vi "Tracking Phaco.vi"(5 "Trajectory Cluster":T3, 6 "OCT Z PID Gains":cluster{"Kp":dbl, "Kd":dbl, "Ki":dbl}={"Kp"=0.0003, "Kd"=0.0001, "Ki"=0.01}, 7 "Eye Model Cluster":T2={"X Grid"=[], "Y Grid"=[], "Za_true Surf"=[], "Iris Center"=[], "Zp_true Surf"=[], "Pinv"=[[1.0, 0.0], [0.0, 1.0]], "za_true"=5.0, "za_work"=1.0, "zp_work"=-1.0, "zp_true"=-5.0}, 8 "error in":errorcluster, 9 "OCT Prev Posit":dbl, 10 "Resume Index":i32, 11 "FPGA VI Reference In":refnum<k20>) -> (0 "error out":errorcluster, 1 "OCT Last Posit":dbl, 2 "Leave Index":i32, 3 "FPGA VI Reference Out":refnum<k20>)   [LabVIEW 2016]
uses:
  <vilib>/Analysis/Matrix/Datatypes/RealMatrix.ctl
  <vilib>/Platform/TimedLoop/XDataNode/timing_clust.ctl
  <vilib>/Platform/TimedLoop/XDataNode/nitl_modes.ctl
  <vilib>/Platform/TimedLoop/XDataNode/wakeup.ctl
  Subsystems/Global Variables.vi
  <vilib>/platform/TimedLoop/XDataNode/XDataNode.xnode
  <vilib>/Platform/TimedLoop/XDataNode/XDNodeRunTimeDep.lvlib
  Library/KevinLibraryAll/labview/KevLib01.lvlib
  <vilib>/Analysis/Matrix/NI_Matrix.lvlib
panel:
  out "In Servo Loop":bool
  out "PC z Displacement":dbl
  out "Speed Schedule":dbl
  out "joint limits":dbl[][](array[numeric])=[[-10.0, 35.0], [-35.0, 35.0], [0.1, 10.0], [-40.0, 40.0]]
  out "Vac Extremum":dbl[](array[numeric])
  out "z Dist Thld":dbl[](array[numeric])
  out "z Rot Axis":dbl
  out "Deform Array":dbl[](array[numeric])=[1.0, 1.0, 1.0, 0.0, 0.0, 0.0, 0.0, 0.0, 0.0]
  out "Speed Override":u16(ring)=3 items=["4x", "3x", "2x", "1x", "0.5x", "0.2x", "0.1x", "PAUSE"]
  out "Loading Finished":bool
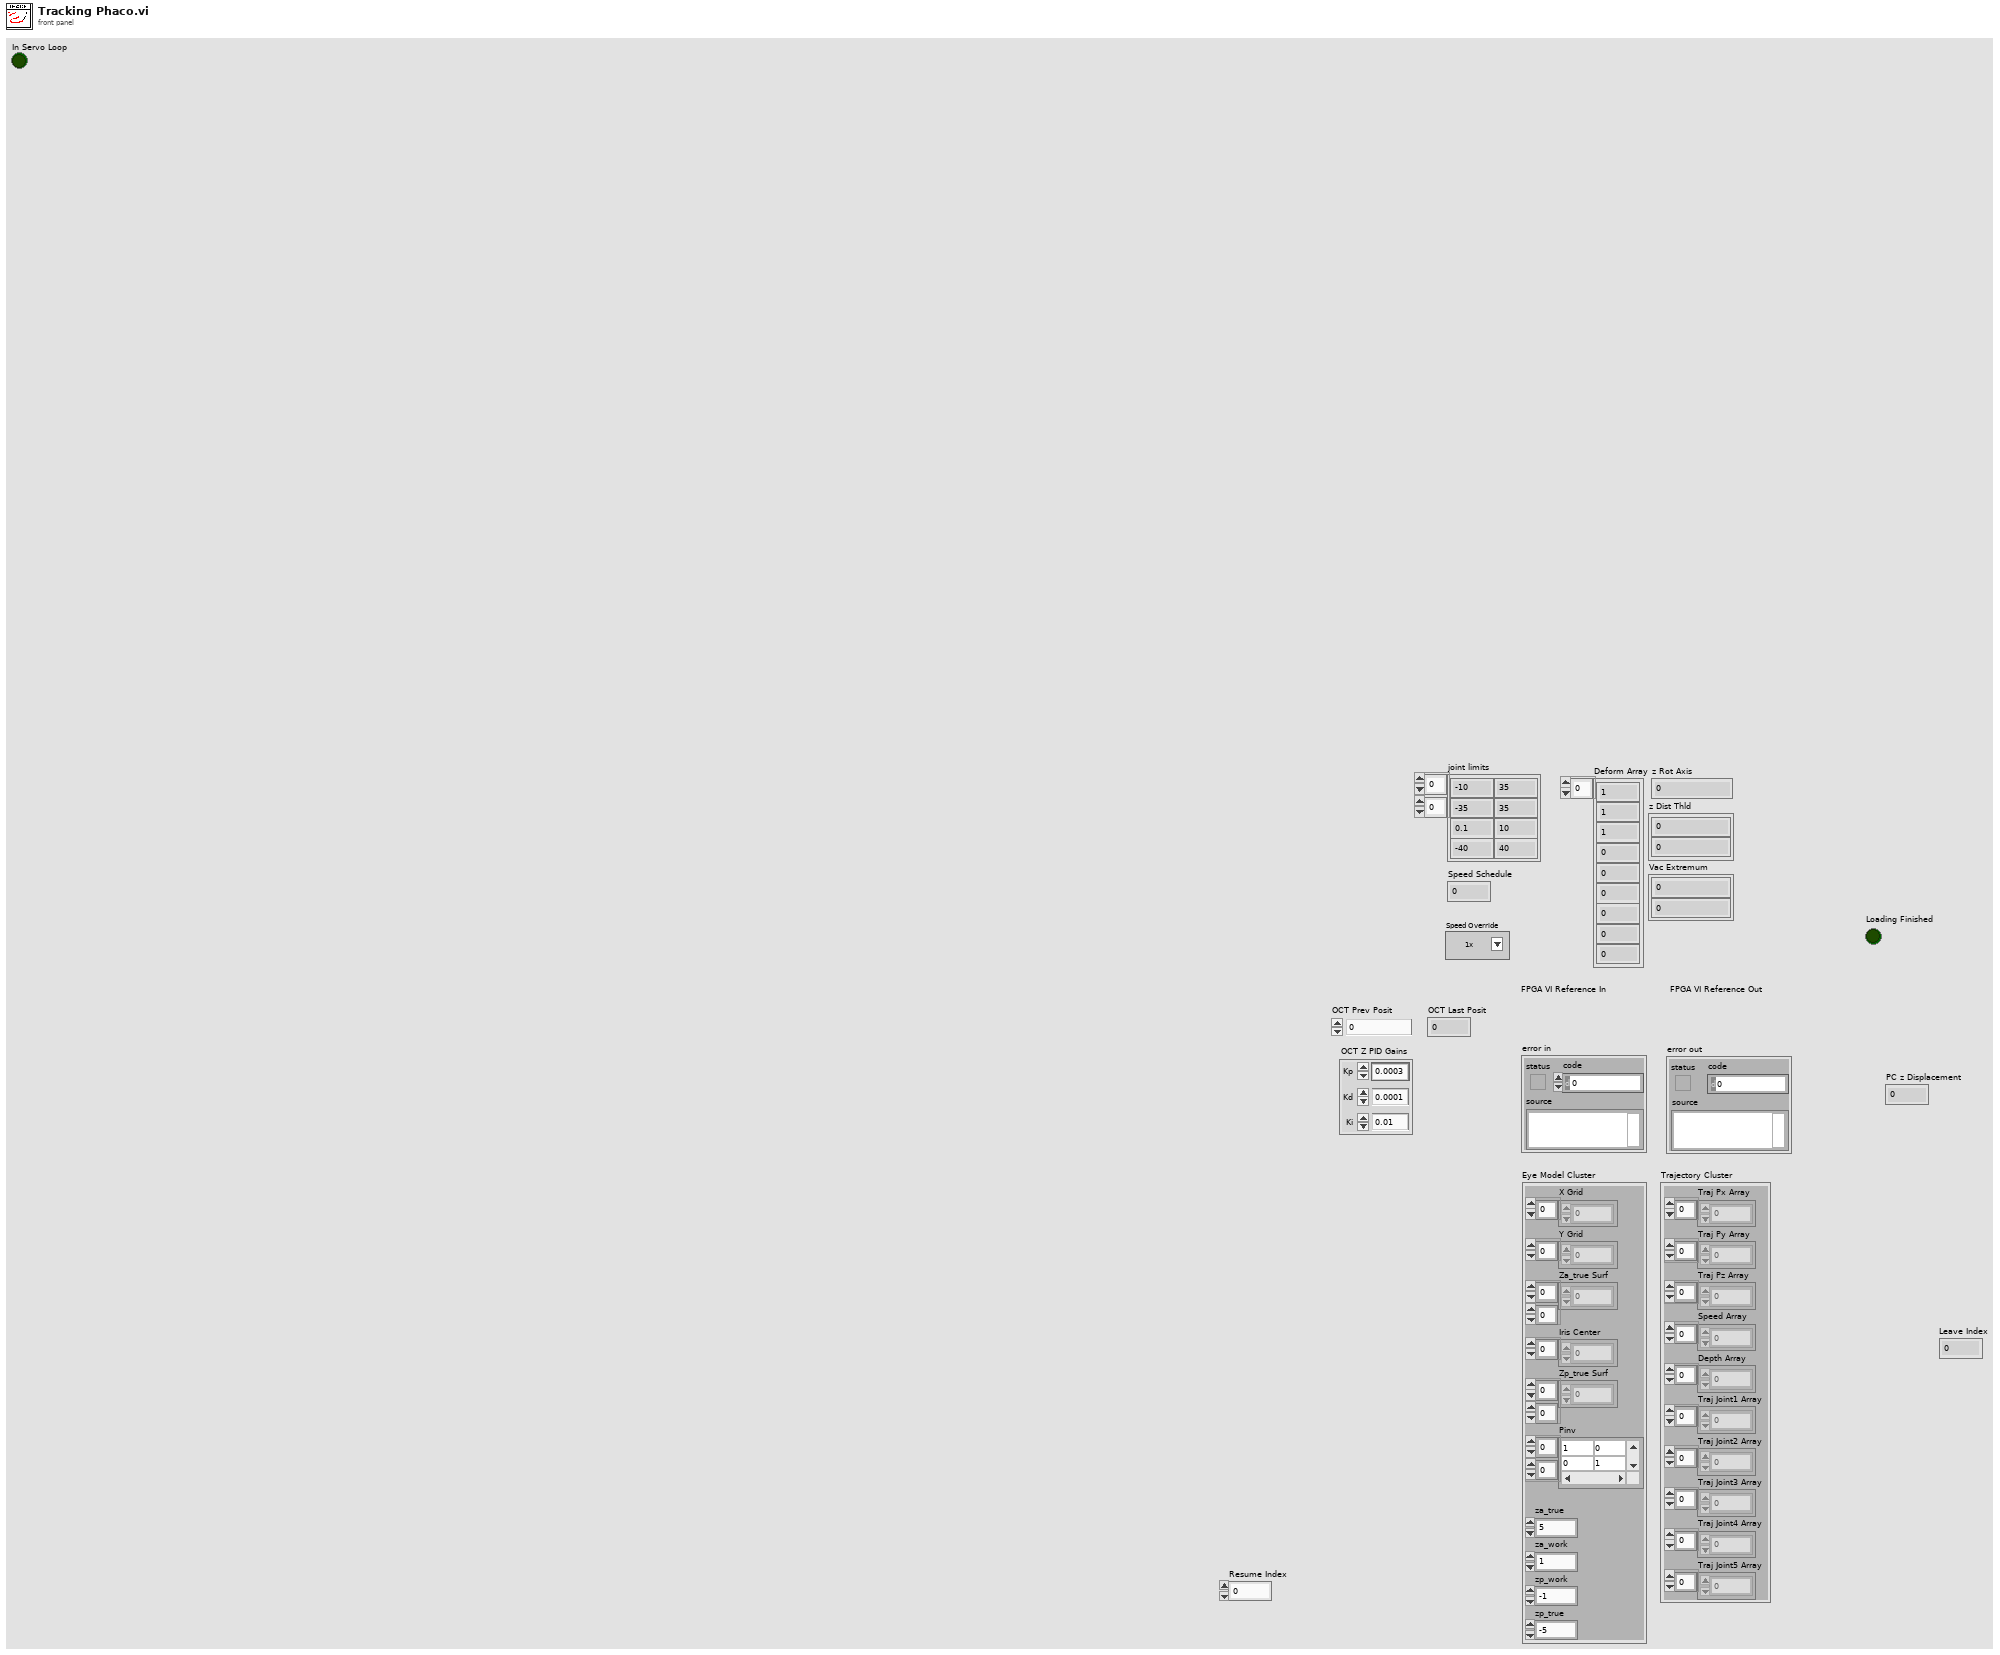
[diagram p1: front panel]
types:
  T1 = typedef "NI_Matrix.lvlib/RealMatrix.ctl" = dbl[][]
  T2 = cluster{"X Grid":dbl[], "Y Grid":dbl[], "Za_true Surf":dbl[][], "Iris Center":dbl[], "Zp_true Surf":dbl[][], "Pinv":T1, "za_true":dbl, "za_work":dbl, "zp_work":dbl, "zp_true":dbl}
  T3 = cluster{"Traj Px Array":dbl[], "Traj Py Array":dbl[], "Traj Pz Array":dbl[], "Speed Array":dbl[], "Depth Array":dbl[], "Traj Joint1 Array":dbl[], "Traj Joint2 Array":dbl[], "Traj Joint3 Array":dbl[], "Traj Joint4 Array":dbl[], "Traj Joint5 Array":dbl[]}
  T4 = typedef "XDNodeRunTimeDep.lvlib/timing_clust.ctl" = cluster{"Expected End [f-1]":u64, "Actual End [f-1]":u64, "Finished Late? [f-1]":bool, "Expected End [i-1]":u64, "Actual End [i-1]":u64, "Finished Late? [i-1]":bool, "Expected Start [i]":u64, "Actual Start [i]":u64, "Expected Start [f]":u64, "Actual Start [f]":u64, "Source Name":string, "Structure Name":string, "Period":i64, "Deadline":i64, "Offset":i64, "Start":i64, "Priority":i32, "Timeout":i32, "Mode":T5, "Wakeup Reason":T6, "Error":errorcluster, "Source Type":string, "Secondary Source Type":string, "Global End Time":u64, "Global Start Time":u64, "Frame Duration":u64, "Iteration Duration":u64, "Assigned CPU":i32, "I/O Scan Engine Mode":u32}
  T5 = typedef "XDNodeRunTimeDep.lvlib/nitl_modes.ctl" = enum32{"No Change", "Process missed periods, maintain original phase", "Discard missed periods, maintain original phase", "Process missed periods, ignore original phase", "Discard missed periods, ignore original phase"}
  T6 = typedef "XDNodeRunTimeDep.lvlib/wakeup.ctl" = enum32{"Normal", "Aborted", "Asynchronous wakeup", "Timing source error", "Timed loop error", "Timeout"}
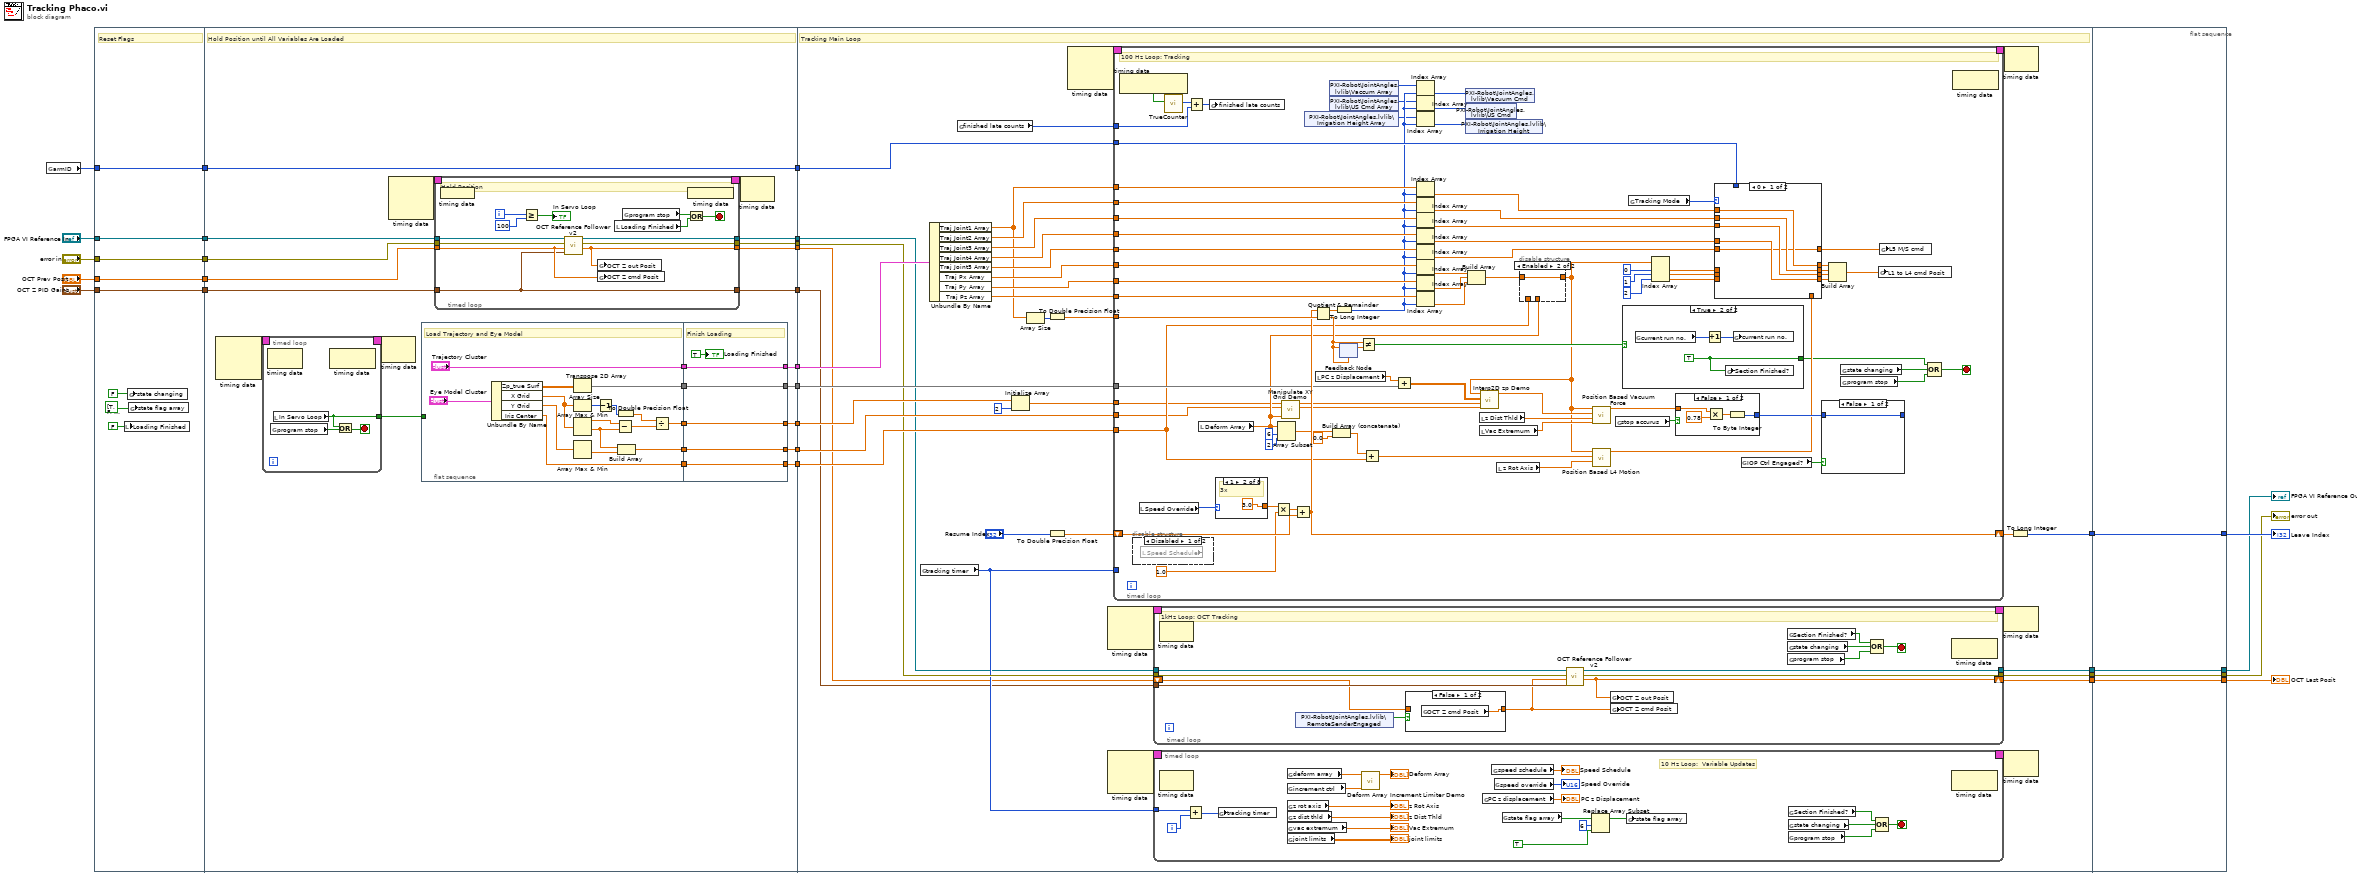
[diagram p0: block diagram]
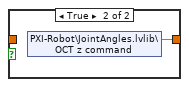
[diagram p2: hidden frame]
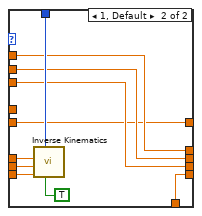
[diagram p3: hidden frame]
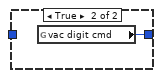
[diagram p5: hidden frame]
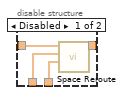
[diagram p6: hidden frame]
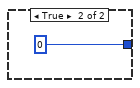
[diagram p7: hidden frame]
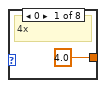
[diagram p8: hidden frame]
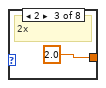
[diagram p9: hidden frame]
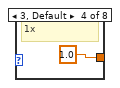
[diagram p10: hidden frame]
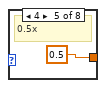
[diagram p11: hidden frame]
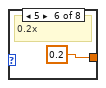
[diagram p12: hidden frame]
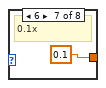
[diagram p13: hidden frame]
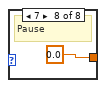
[diagram p14: hidden frame]
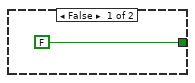
[diagram p15: hidden frame]
diagram:
  n1 = global read "Global Variables.vi" "armID"() -> (w14:i32)
  n2 = flat-sequence {
    tunnel: [w34] -> w28
    tunnel: "FPGA VI Reference In" -> [w34]
    tunnel: "error in" -> [w33]
    tunnel: [w33] -> w25
    tunnel: w14 -> [w32]
    tunnel: [w32] -> w16
    tunnel: [w30] -> w13
    tunnel: "OCT Prev Posit" -> [w30]
    tunnel: [w29] -> w11
    tunnel: "OCT Z PID Gains" -> [w29]
    tunnel: w28 -> [w47]
    tunnel: w25 -> [w46]
    tunnel: [w42] -> w24
    tunnel: [w60] -> w23
    tunnel: [w59] -> w22
    tunnel: [w58] -> w21
    tunnel: [w57] -> w19
    tunnel: [w56] -> w18
    tunnel: [w50] -> w17
    tunnel: w16 -> [w50]
    tunnel: [w43] -> w15
    tunnel: w13 -> [w45]
    tunnel: w11 -> [w44]
    tunnel: [w38] -> w9
    tunnel: [w37] -> w8
    tunnel: w24 -> [w123]
    tunnel: w23 -> [w137]
    tunnel: w22 -> [w129]
    tunnel: w21 -> [w138]
    tunnel: w19 -> [w130]
    tunnel: w18 -> [w131]
    tunnel: w17 -> [w126]
    tunnel: w15 -> [w120]
    tunnel: w9 -> [w119]
    tunnel: w8 -> [w118]
    tunnel: [w134] -> w6
    tunnel: [w122] -> w5
    tunnel: [w117] -> w4
    tunnel: [w107] -> w3
    tunnel: [w315] -> w7
    tunnel: [w316] -> w1
    tunnel: [w317] -> w20
    tunnel: w6 -> [w317]
    tunnel: w5 -> [w316]
    tunnel: w4 -> [w315]
    tunnel: w3 -> [w314]
    tunnel: [w314] -> w2
    frame #0 {
      # "Reset Flags"
      n3 = local write "Loading Finished"(FALSE ("Loading Finished")) -> ()
      n4 = global write "Global Variables.vi" "state changing"(FALSE ("state changing")) -> ()
      n5 = global write "Global Variables.vi" "state flag array"(bool[] [TRUE, FALSE, FALSE, FALSE, FALSE, FALSE, FALSE, FALSE, FALSE] ("state flag array")) -> ()
    }
    frame #1 {
      # "Hold Position until All Variables Are Loaded"
      n6 = node-c288() -> (w41:T4)  [unwired: 3 in]
      n7 = timed-loop {
        timing: w41 -> [_]
        timing-out: [_] -> w40
        tunnel: [w61] -> w39
        stop <- w63 stop-if-true
        n8 = node-c288() -> ()  [unwired: 1 in, 1 out]
        n9 = global read "Global Variables.vi" "program stop"() -> (w62:bool)
        n10 = local read "In Servo Loop"() -> (w61:bool)
        n11 = node-c288() -> ()  [unwired: 1 in, 1 out]
        n12 = Or(x=w61, y=w62) -> (x .or. y?=w63:bool)
      }
      n13 = node-c288(w40) -> ()  [unwired: 1 out]
      n14 = node-c288() -> (w49:T4)  [unwired: 3 in]
      n15 = flat-sequence {
        tunnel: [w87] -> w55
        tunnel: [w100] -> w54
        tunnel: [w99] -> w53
        tunnel: [w86] -> w52
        tunnel: ["Trajectory Cluster"] -> w51
        tunnel: w39 -> [_]
        tunnel: [w104] -> w58
        tunnel: [w105] -> w59
        tunnel: [w106] -> w60
        tunnel: w55 -> [w106]
        tunnel: w54 -> [w105]
        tunnel: w53 -> [w104]
        tunnel: w52 -> [w102]
        tunnel: [w102] -> w57
        tunnel: [w101] -> w56
        tunnel: w51 -> [w101]
        frame #0 {
          # "Load Trajectory and Eye Model"
          n16 = Unbundle By Name("Eye Model Cluster") -> ("Zp_true Surf"=w88:dbl[][], "X Grid"=w89:dbl[], "Y Grid"=w98:dbl[], "Iris Center"=w86:dbl[])
          n17 = Transpose 2D Array(2D array=w88) -> (transposed array=w87:dbl[][])
          n18 = Array Size(array=w89) -> (size(s)=w97:i32)
          n19 = Array Max & Min(array=w89) -> (max value=w95:dbl, min value=w96:dbl)  [unwired: 2 out]
          n20 = Array Max & Min(array=w98) -> (min value=w94:dbl)  [unwired: 3 out]
          n21 = Decrement(x=w97) -> (x-1=w92:i32)
          n22 = Subtract(x=w95, y=w96) -> (x-y=w91:dbl)
          n23 = To Double Precision Float(number=w92) -> (double precision float=w93:dbl)
          n24 = Build Array(w96, w94) -> (w99:dbl[])
          n25 = Divide(x=w93, y=w91) -> (x/y=w100:dbl)
        }
        frame #1 {
          # "Finish Loading"
          "Loading Finished" <- TRUE ("Loading Finished")
        }
      }
      n26 = timed-loop {
        timing: w49 -> [_]
        timing-out: [_] -> w48
        tunnel: [w71] -> w37
        tunnel: [w68] -> w43
        tunnel: [w72] -> w42
        tunnel: w47 -> [w74]
        tunnel: w46 -> [w73]
        tunnel: w44 -> [w69]
        tunnel: w45 -> [w70]
        tunnel: [w69] -> w38
        i -> [w77]
        stop <- w80 stop-if-true
        # "Hold Position"
        n27 = node-c288 ("Output Node")() -> ()  [unwired: 1 in]
        n28 = Greater Or Equal?(x=w77, y=100) -> (x >= y?=→"In Servo Loop":bool)
        n29 = call "OCT Reference Follower v2.vi"("OCT Z PID Gains"=w69, "OCT  Z cmd Posit [mm]"=w70, "error in"=w73, "FPGA VI Reference In"=w74) -> ("OCT  Z out Posit [mm]"=w71:dbl, "error out"=w72:errorcluster, "FPGA VI Reference Out"=w68:refnum<k20>)  [unwired: 5 in]
        n30 = global write "Global Variables.vi" "OCT Z out Posit"(w71) -> ()
        n31 = global write "Global Variables.vi" "OCT Z cmd Posit"(w70) -> ()
        n32 = local read "Loading Finished"() -> (w79:bool)
        n33 = global read "Global Variables.vi" "program stop"() -> (w78:bool)
        n34 = Or(x=w78, y=w79) -> (x .or. y?=w80:bool)
        n35 = node-c288() -> ()  [unwired: 1 out]
      }
      n36 = node-c288(w48) -> ()  [unwired: 1 out]
    }
    frame #2 {
      # "Tracking Main Loop"
      n37 = global read "Global Variables.vi" "tracking timer"() -> (w121:i32)
      n38 = Unbundle By Name(w131) -> ("Traj Joint1 Array"=w110:dbl[], "Traj Joint2 Array"=w116:dbl[], "Traj Joint3 Array"=w115:dbl[], "Traj Joint4 Array"=w114:dbl[], "Traj Joint5 Array"=w111:dbl[], "Traj Px Array"=w113:dbl[], "Traj Py Array"=w136:dbl[], "Traj Pz Array"=w132:dbl[])
      n39 = global read "Global Variables.vi" "finished late counts"() -> (w141:u16)
      n40 = Initialize Array(w129, 2 ("dimension size")) -> (w127:dbl[])
      n41 = Array Size(array=w110) -> (size(s)=w109:i32)
      n42 = To Double Precision Float(number=w109) -> (double precision float=w112:dbl)
      n43 = To Double Precision Float(number="Resume Index") -> (double precision float=w133:dbl)
      n44 = node-c288() -> (w143:T4)  [unwired: 3 in]
      n45 = node-c288() -> (w125:T4)  [unwired: 3 in]
      n46 = node-c288() -> (w140:T4)  [unwired: 3 in]
      n47 = timed-loop {
        timing: w143 -> [_]
        timing-out: [_] -> w142
        tunnel: w113 -> [w269]
        tunnel: w136 -> [w268]
        tunnel: w132 -> [w263]
        tunnel: w141 -> [w264]
        shift-right: [w250] -> w135
        shift-left: w133 -> [w253]
        tunnel: w137 -> [w246]
        tunnel: w127 -> [w243]
        tunnel: w138 -> [w242]
        tunnel: w112 -> [w252]
        tunnel: w130 -> [w245]
        tunnel: w121 -> [_]
        tunnel: w126 -> [w213]
        tunnel: w110 -> [w210]
        tunnel: w116 -> [w211]
        tunnel: w115 -> [w212]
        tunnel: w114 -> [w203]
        tunnel: w111 -> [w202]
        stop <- w196 stop-if-true
        # "100 Hz Loop: Tracking"
        n48 = node-c288() -> (w267:bool)  [unwired: 1 in]
        n49 = disable-structure shown="Disabled" {
          frame Disabled {
            n50 = local read "Speed Schedule"() -> ()  [unwired: 1 out]
          }
          frame Enabled {
          }
        }
        n51 = local read "Speed Override"() -> (w255:u16)
        n52 = call "TrueCounter.vi"("True?"=w267) -> ("True Count"=w265:u16)  [unwired: 10 in]
        n53 = Add(x=w265, y=w264) -> (x+y=w266:u16)
        n54 = local read "Deform Array"() -> (w244:dbl[])
        n55 = global write "Global Variables.vi" "finished late counts"(w266) -> ()
        n56 = case shown="1" w255 {
          tunnel: [4.0 ("y") 3.0 ("y") 2.0 ("y") 1.0 ("y") 0.5 ("y") 0.2 ("y") 0.1 ("y") 0.0 ("y")] -> w254
          frame 0 {
            # "4x"
          }
          frame 1 {
            # "3x"
          }
          frame 2 {
            # "2x"
          }
          frame 3, Default {
            # "1x"
          }
          frame 4 {
            # "0.5x"
          }
          frame 5 {
            # "0.2x"
          }
          frame 6 {
            # "0.1x"
          }
          frame 7 {
            # "Pause"
          }
        }
        n57 = Multiply(x=w254, y=1.0) -> (x*y=w256:dbl)
        n58 = Array Subset(array=w244, index=6, length=2) -> (w229:dbl[])
        n59 = call "Manipulate XY Grid Demo.vi"("Deform Array"=w244, "XY Grid min In"=w242, "XY Quant. Fact. In"=w243) -> ("XY Grid min Out"=w224:dbl[], "XY Quant. Fact. Out"=w225:dbl[])  [unwired: 7 in]
        n60 = Add(x=w256, y=w253) -> (x+y=w250:dbl)
        n61 = shared-variable "PXI-Robot\\JointAngles.lvlib\\Irrigation Height Array"() -> (w194:i32[])  [unwired: 1 in, 1 out]
        n62 = Quotient & Remainder(x=w250, y=w252) -> (x-y*floor(x/y)=w251:dbl, floor(x/y)=w247:dbl)
        n63 = local read "PC z Displacement"() -> (w232:dbl)
        n64 = shared-variable "PXI-Robot\\JointAngles.lvlib\\Vaccum Array"() -> (w193:i32[])  [unwired: 1 in, 1 out]
        n65 = shared-variable "PXI-Robot\\JointAngles.lvlib\\US Cmd Array"() -> (w192:i32[])  [unwired: 1 in, 1 out]
        n66 = Build Array (concatenate)(w229, 0.0) -> (w228:dbl[])
        n67 = To Long Integer(number=w251) -> (32bit integer=w195:i32)
        n68 = feedback-in #1(w247) -> ()
        n69 = feedback #1(w247) -> (w249:dbl)
        n70 = Not Equal?(x=w247, y=w249) -> (x != y?=w248:bool)
        n71 = Add(x=w228, y=w245) -> (x+y=w219:dbl[])
        n72 = Add(x=w232, y=w246) -> (x+y=w226:dbl[][])
        n73 = Index Array(array=w193, index=w195) -> (element=w189:i32)
        n74 = Index Array(array=w192, index=w195) -> (element=w191:i32)
        n75 = Index Array(array=w194, index=w195) -> (element=w190:i32)
        n76 = Index Array(array=w210, index=w195) -> (element=w208:dbl)
        n77 = Index Array(array=w211, index=w195) -> (element=w207:dbl)
        n78 = Index Array(array=w212, index=w195) -> (element=w206:dbl)
        n79 = Index Array(array=w203, index=w195) -> (element=w201:dbl)
        n80 = Index Array(array=w202, index=w195) -> (element=w200:dbl)
        n81 = Index Array(array=w269, index=w195) -> (element=w259:dbl)
        n82 = Index Array(array=w268, index=w195) -> (element=w258:dbl)
        n83 = Index Array(array=w263, index=w195) -> (element=w257:dbl)
        n84 = shared-variable "PXI-Robot\\JointAngles.lvlib\\Vacuum Cmd"(w189) -> ()  [unwired: 1 in, 1 out]
        n85 = shared-variable "PXI-Robot\\JointAngles.lvlib\\US Cmd"(w191) -> ()  [unwired: 1 in, 1 out]
        n86 = shared-variable "PXI-Robot\\JointAngles.lvlib\\Irrigation Height"(w190) -> ()  [unwired: 1 in, 1 out]
        n87 = Build Array(w259, w258, w257) -> (w241:dbl[])
        n88 = local read "z Dist Thld"() -> (w222:dbl[])
        n89 = local read "Vac Extremum"() -> (w221:dbl[])
        n90 = local read "z Rot Axis"() -> (w218:dbl)
        n91 = disable-structure shown="Enabled" {
          disable-tunnel: w245 -> [w290 _]
          disable-tunnel: w244 -> [w289 _]
          disable-tunnel: w241 -> [w288 w291]
          disable-tunnel: [w287 w291] -> w217
          frame Disabled {
            n92 = call "Space Reroute.vi"("Deform Array"=w289, "Pivot Pt"=w290, "Nominal Traj Pt"=w288) -> ("Reroute Traj Pt"=w287:dbl[])  [unwired: 8 in]
          }
          frame Enabled {
          }
        }
        n93 = call "Interp2D zp Demo.vi"("XY Grid min"=w224, "XY Quantization Factor"=w225, "Zp array"=w226, "Tip Position"=w217) -> ("zp"=w223:dbl)  [unwired: 7 in]
        n94 = call "Position Based Vacuum Force.vi"("vac_bnd"=w221, "z_thld"=w222, "current zp"=w223, "tip position"=w217) -> ("vacf (%)"=w220:dbl)  [unwired: 7 in]
        n95 = call "Position Based L4 Motion.vi"("Assign z"=w218, "Iris Center"=w219, "Tip Position"=w217) -> ("L4 Motion [deg]"=w205:dbl)  [unwired: 8 in]
        n96 = global read "Global Variables.vi" "stop accurus"() -> (w233:bool)
        n97 = case shown="True" w248 {
          tunnel: [FALSE ("Section Finished?") w306] -> w188
          frame False {
          }
          frame True {
            w306 = TRUE ("Section Finished?")
            n98 = global read "Global Variables.vi" "current run no."() -> (w308:u8)
            n99 = Increment(x=w308) -> (x+1=w307:u8)
            n100 = global write "Global Variables.vi" "Section Finished?"(w306) -> ()
            n101 = global write "Global Variables.vi" "current run no."(w307) -> ()
          }
        }
        n102 = global read "Global Variables.vi" "Tracking Mode"() -> (w209:u16)
        n103 = Index Array(array=w217, index #1=0 ("index"), index #2=1 ("index"), index #3=2 ("index")) -> (element #1=w240:dbl, element #2=w239:dbl, element #3=w238:dbl)
        n104 = case shown="False" w233 {
          tunnel: w220 -> [w293 _]
          tunnel: [w292 i8 0 ("Digital Cmd [0-78]")] -> w215
          frame False {
            n105 = Multiply(x=w293, y=0.78 ("x")) -> (x*y=w294:dbl)
            n106 = To Byte Integer(number=w294) -> (8bit integer=w292:i8)
          }
          frame True {
          }
        }
        n107 = case shown="0" w209 {
          tunnel: w240 -> [_ w283]
          tunnel: w239 -> [_ w282]
          tunnel: w238 -> [_ w281]
          tunnel: [w274 w278] -> w237
          tunnel: [w273 w277] -> w236
          tunnel: [w272 w276] -> w235
          tunnel: w213 -> [_ w280]
          tunnel: w208 -> [w274 w278]
          tunnel: w207 -> [w273 w277]
          tunnel: w206 -> [w272 w276]
          tunnel: w205 -> [_ w279]
          tunnel: [w271 w279] -> w204
          tunnel: w201 -> [w271 _]
          tunnel: w200 -> [w270 w275]
          tunnel: [w270 w275] -> w199
          frame 0 {
          }
          frame 1, Default {
            n108 = call "Inverse Kinematics.vi"("isToolTipInsideEye"=TRUE, "armID"=w280, "z"=w281, "y"=w282, "x"=w283) -> ()  [unwired: 3 in, 4 out]
          }
        }
        n109 = global read "Global Variables.vi" "IOP Ctrl Engaged?"() -> (w216:bool)
        n110 = case shown="False" w216 {
          tunnel: [w285 w286] -> _
          tunnel: w215 -> [w285 _]
          frame False {
          }
          frame True {
            n111 = global read "Global Variables.vi" "vac digit cmd"() -> (w286:i8)
          }
        }
        n112 = Build Array(w237, w236, w235, w204) -> (w234:dbl[])
        n113 = global read "Global Variables.vi" "state changing"() -> (w198:bool)
        n114 = global read "Global Variables.vi" "program stop"() -> (w197:bool)
        n115 = global write "Global Variables.vi" "L1 to L4 cmd Posit"(w234) -> ()
        n116 = global write "Global Variables.vi" "L5 M/S cmd"(w199) -> ()
        n117 = Compound Arithmetic op=OR(w188, w198, w197) -> (w196:bool)
        n118 = node-c288() -> ()  [unwired: 1 in, 1 out]
      }
      n119 = timed-loop {
        timing: w125 -> [_]
        timing-out: [_] -> w124
        tunnel: w123 -> [w156]
        tunnel: [w155] -> w122
        tunnel: w120 -> [w154]
        tunnel: w119 -> [w153]
        shift-right: [w149] -> w117
        shift-left: w118 -> [w151]
        tunnel: [w145] -> w107
        stop <- w146 stop-if-true
        # "1kHz Loop: OCT Tracking"
        n120 = node-c288() -> ()  [unwired: 1 in, 1 out]
        n121 = shared-variable "PXI-Robot\\JointAngles.lvlib\\RemoteSenderEngaged"() -> (w152:bool)  [unwired: 1 in, 1 out]
        n122 = case shown="False" w152 {
          tunnel: [w157 w158] -> w150
          tunnel: w151 -> [_ _]
          frame False {
            # "Hold Position if not Engaged"
            n123 = global read "Global Variables.vi" "OCT Z cmd Posit"() -> (w157:dbl)
          }
          frame True {
            n124 = shared-variable "PXI-Robot\\JointAngles.lvlib\\OCT z command"() -> (w158:dbl)  [unwired: 1 in, 1 out]
          }
        }
        n125 = call "OCT Reference Follower v2.vi"("OCT Z PID Gains"=w153, "OCT  Z cmd Posit [mm]"=w150, "error in"=w156, "FPGA VI Reference In"=w154) -> ("OCT  Z out Posit [mm]"=w149:dbl, "error out"=w155:errorcluster, "FPGA VI Reference Out"=w145:refnum<k20>)  [unwired: 5 in]
        n126 = global write "Global Variables.vi" "OCT Z out Posit"(w149) -> ()
        n127 = global write "Global Variables.vi" "OCT Z cmd Posit"(w150) -> ()
        n128 = global read "Global Variables.vi" "Section Finished?"() -> (w144:bool)
        n129 = global read "Global Variables.vi" "state changing"() -> (w148:bool)
        n130 = global read "Global Variables.vi" "program stop"() -> (w147:bool)
        n131 = Compound Arithmetic op=OR(w144, w148, w147) -> (w146:bool)
        n132 = node-c288() -> ()  [unwired: 1 in, 1 out]
      }
      n133 = timed-loop {
        timing: w140 -> [_]
        timing-out: [_] -> w139
        tunnel: w121 -> [w170]
        i -> [w171]
        stop <- w164 stop-if-true
        # "10 Hz Loop:  Variable Updates"
        n134 = node-c288() -> ()  [unwired: 1 in, 1 out]
        n135 = Add(x=w170, y=w171) -> (x+y=w172:i32)
        n136 = global write "Global Variables.vi" "tracking timer"(w172) -> ()
        n137 = global read "Global Variables.vi" "deform array"() -> (w169:dbl[])
        n138 = global read "Global Variables.vi" "increment ctrl"() -> (w168:dbl[])
        n139 = global read "Global Variables.vi" "z rot axis"() -> (→"z Rot Axis":dbl)
        n140 = global read "Global Variables.vi" "z dist thld"() -> (→"z Dist Thld":dbl[])
        n141 = global read "Global Variables.vi" "vac extremum"() -> (→"Vac Extremum":dbl[])
        n142 = global read "Global Variables.vi" "joint limits"() -> (→"joint limits":dbl[][])
        n143 = call "Deform Array Increment Limiter Demo.vi"("Increment Array"=w168, "Defrom Ref"=w169) -> ("Deform Output"=→"Deform Array":dbl[])  [unwired: 9 in]
        n144 = global read "Global Variables.vi" "PC z displacement"() -> (→"PC z Displacement":dbl)
        n145 = global read "Global Variables.vi" "speed schedule"() -> (→"Speed Schedule":dbl)
        n146 = global read "Global Variables.vi" "speed override"() -> (→"Speed Override":u16)
        n147 = global read "Global Variables.vi" "state flag array"() -> (w175:bool[])
        n148 = Replace Array Subset(array=w175, new element=TRUE ("new element/subarray"), index=6) -> (w176:bool[])
        n149 = global write "Global Variables.vi" "state flag array"(w176) -> ()
        n150 = global read "Global Variables.vi" "Section Finished?"() -> (w163:bool)
        n151 = global read "Global Variables.vi" "state changing"() -> (w166:bool)
        n152 = global read "Global Variables.vi" "program stop"() -> (w165:bool)
        n153 = Compound Arithmetic op=OR(w163, w166, w165) -> (w164:bool)
        n154 = node-c288() -> ()  [unwired: 1 in, 1 out]
      }
      n155 = node-c288(w124) -> ()  [unwired: 1 out]
      n156 = node-c288(w139) -> ()  [unwired: 1 out]
      n157 = node-c288(w142) -> ()  [unwired: 1 out]
      n158 = To Long Integer(number=w135) -> (32bit integer=w134:i32)
    }
    frame #3 {
    }
  }
  "FPGA VI Reference Out" <- w2
  "error out" <- w1
  "Leave Index" <- w20
  "OCT Last Posit" <- w7
